vi "Check Cluster Configuration Store.vi"(8 "error in (no error)":errorcluster, 10 "register name":string, 11 "Cluster Configuration Store in":T3) -> (0 "error IO":errorcluster, 1 "Found":bool, 2 "Cluster Configuration out":T1, 3 "Cluster Configuration Store out":T3)   [LabVIEW 2018, in "Scalar IO Operations.lvlib"]
uses:
  Scalar IO Operations.lvlib
  TypeDefs/Cluster Configuration Store.ctl
  TypeDefs/Cluster Configuration.ctl
  <vilib>/Utility/Data Type/Type Definitions/Data Type.ctl
  <vilib>/Utility/Data Type/NI_Data Type.lvlib
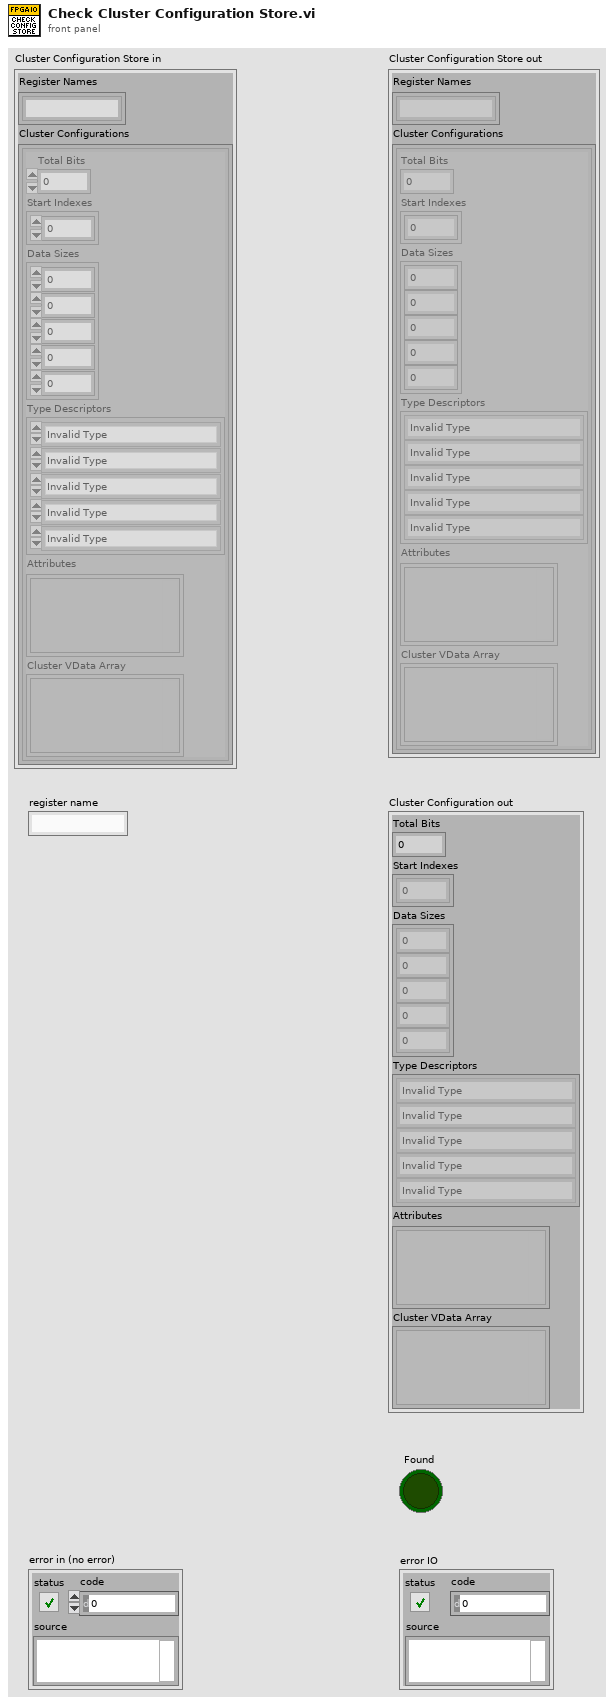
[diagram p1: front panel]
types:
  T1 = typedef "Scalar IO Operations.lvlib/Cluster Configuration.ctl" = cluster{"Total Bits":i32, "Start Indexes":i32[], "Data Sizes":i32[], "Type Descriptors":T2[], "Attributes":variant[], "Cluster VData Array":variant[]}
  T2 = typedef "NI_Data Type.lvlib/Data Type.ctl" = enum8{"Invalid Type", "Void", "I8", "I16", "I32", "I64", "U8", "U16", "U32", "U64", "Single Float", "Double Float", "Extended Float", "Single Complex", "Double Complex", "Extended Complex", "Enum U8", "Enum U16", "Enum U32", "Enum U64", "Single Float With Unit", "Double Float With Unit", "Extended Float With Unit", "Single Complex with Unit", "Double Complex with Unit", "Extended Complex with Unit", "Boolean", "String", "Path", "Picture", "Tag", "Array", "Cluster", "Variant", "LV Variant", "Waveform", "Timestamp", "Digital Waveform", "Digital Data", "ExpressData", "Refnum", "External Data", "VI", "Poly VI", "LabVIEW Class Instance", "Fixed Point"}
  T3 = typedef "Scalar IO Operations.lvlib/Cluster Configuration Store.ctl" = cluster{"Register Names":string[], "Cluster Configurations":T1[]}
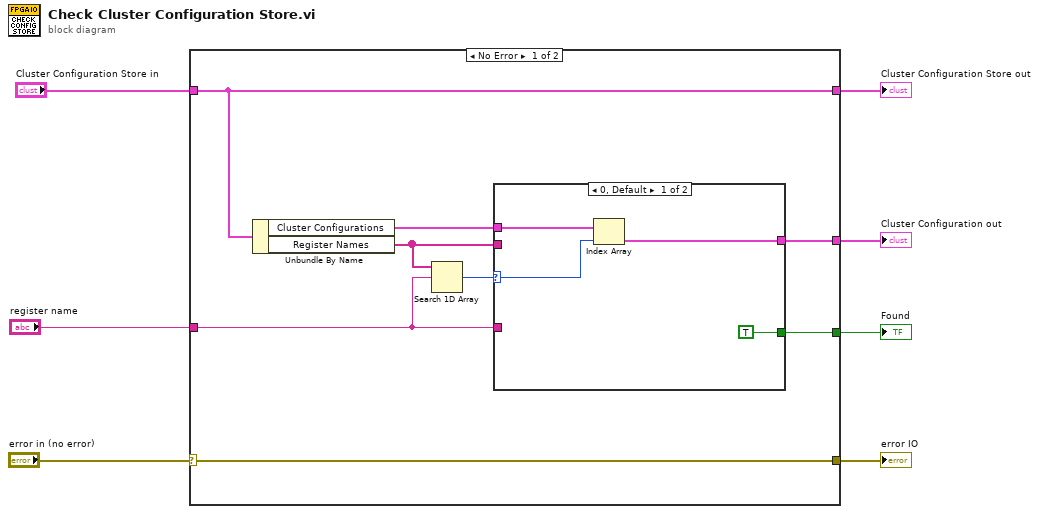
[diagram p0: block diagram]
diagram:
  n1 = case shown="No Error" "error in (no error)" {
    selector: "error in (no error)" -> [w8 w21]
    tunnel: "register name" -> [w15 _]
    tunnel: "Cluster Configuration Store in" -> [w9 w20]
    tunnel: [w11 _] -> w1
    tunnel: [w10 _] -> w6
    tunnel: [w9 w20] -> w2
    tunnel: [w8 w21] -> w4
    frame No Error {
      n2 = Unbundle By Name(w9) -> ("Cluster Configurations"=w14:T1[], "Register Names"=w13:string[])
      n3 = Search 1D Array(1D array=w13, element=w15) -> (index of element=w12:i32)  [unwired: 1 in]
      n4 = case shown="0, Default" w12 {
        selector: w12 -> [w18 _]
        tunnel: w13 -> [_ _]
        tunnel: w14 -> [w19 _]
        tunnel: [w17 _] -> w11
        tunnel: w15 -> [_ _]
        tunnel: [TRUE _] -> w10
        frame 0, Default {
          n5 = Index Array(array=w19, index=w18) -> (element=w17:T1)
        }
        frame -1 {
        }
      }
    }
    frame Error {
    }
  }
  "Found" <- w6
  "error IO" <- w4
  "Cluster Configuration Store out" <- w2
  "Cluster Configuration out" <- w1
